vi "P2_3_TanqueAgua.vi"() -> ()   [LabVIEW 2020]
panel:
  out "Termometro 3":dbl(slide) scale=25.0..100.0
  out "proceos finalizado":bool
  out "Tanke":dbl(slide) scale=0.0..100.0
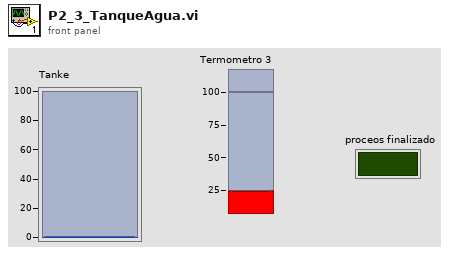
[diagram p1: front panel]
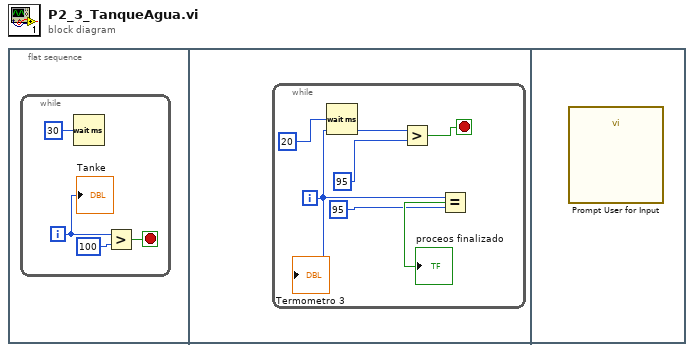
[diagram p0: block diagram]
diagram:
  n1 = flat-sequence {
    frame #0 {
    }
    frame #1 {
      n2 = while {
        i -> [w3]
        stop <- w1 stop-if-true
        n3 = Wait (ms)(milliseconds to wait=u32 20) -> ()  [unwired: 1 out]
        n4 = Greater?(x=w3, y=95) -> (0:w1:bool)
        n5 = Equal?(x=w3, y=95) -> (x = y?=→"proceos finalizado":bool)
        "Termometro 3" <- w3
      }
    }
    frame #2 {
      n6 = call "Prompt User for Input"() -> ()  [unwired: 18 in, 2 out]
    }
  }
  n7 = while {
    i -> [w8]
    stop <- w9 stop-if-true
    n8 = Wait (ms)(milliseconds to wait=u32 30) -> ()  [unwired: 1 out]
    n9 = Greater?(x=w8, y=100) -> (0:w9:bool)
    "Tanke" <- w8
  }
